vi "GetControlRefFromControlArray.vi"(0 "Controls[]":refnum<vi>[](array[refnum]), 7 "Label Text":string, 11 "error In":errorcluster) -> (4 "Remaining Controls[]":refnum<vi>[](array[refnum]), 8 "Target Control":refnum<vi>, 15 "error out":errorcluster)   [LabVIEW 2016]
uses:
  <vilib>/Utility/error.llb/Error Cluster From Error Code.vi
  <vilib>/ErrorRing/Error Ring.xnode
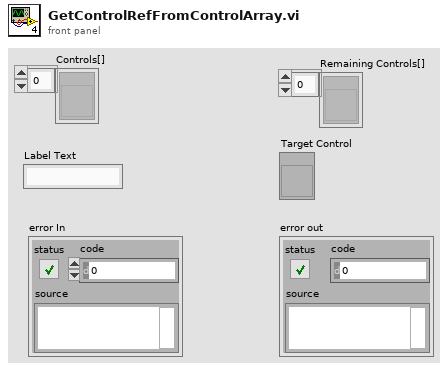
[diagram p1: front panel]
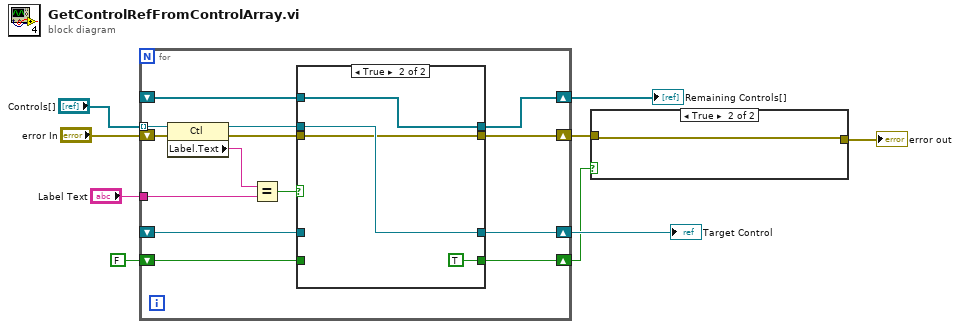
[diagram p0: block diagram]
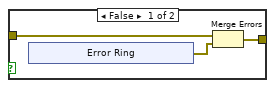
[diagram p2: hidden frame]
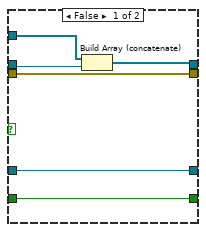
[diagram p3: hidden frame]
diagram:
  n1 = for {
    tunnel: "Controls[]" -> [w23] mode=indexing
    tunnel: "Label Text" -> [w21]
    shift-right: [w18] -> w7
    shift-left: _ -> [w17]
    shift-right: [w16] -> w6
    shift-left: _ -> [w15]
    shift-right: [w13] -> w2
    shift-left: FALSE -> [w14]
    shift-right: [w10] -> w3
    shift-left: "error In" -> [w12]
    n2 = property class="Ctl"(reference=w23, error in=w12) -> (reference out=w19:refnum<vi>, error out=w11:errorcluster, "Label.Text"=w22:string)
    n3 = Equal?(x=w22, y=w21) -> (x = y?=w20:bool)
    n4 = case shown="True" w20 {
      tunnel: w19 -> [w28 w32]
      tunnel: [w27 w33] -> w18
      tunnel: w17 -> [w29 w33]
      tunnel: [w26 w32] -> w16
      tunnel: w15 -> [w26 _]
      tunnel: w14 -> [w25 _]
      tunnel: [w25 TRUE] -> w13
      tunnel: w11 -> [w24 w30]
      tunnel: [w24 w30] -> w10
      frame False {
        n5 = Build Array (concatenate)(w29, w28) -> (w27:refnum<vi>[])
      }
      frame True {
      }
    }
  }
  "Remaining Controls[]" <- w7
  "Target Control" <- w6
  n6 = case shown="True" w2 {
    tunnel: w3 -> [w36 w42]
    tunnel: [w35 w42] -> w1
    frame False {
      n7 = xnode "Error Ring"() -> ("error out"=w34:errorcluster)
      n8 = Merge Errors(w36, w34) -> (w35:errorcluster)
    }
    frame True {
    }
  }
  "error out" <- w1
